vi "PipBoy_SearchLabVIEWs.vi"(8 "error in (no error)":errorcluster, 11 "PipBoyDataIn":T3) -> (0 "error out":errorcluster, 2 "LabVIEWEvents":T1[](array[typedef]), 3 "PipBoyDataOut":T3)   [LabVIEW 2014]
uses:
  ctls/PipBoy_PipBoyData.ctl
  ctls/PipBoy_ProcComm.ctl
  System.Windows.Forms
  ctls/PipBoy_PipBoyCommand.ctl
  ctls/PipBoy_Message.ctl
  modules/support/Message Queue/All Message Queues.ctl
  modules/support/Message Queue/Message Cluster.ctl
  ctls/PipBoy_FileConf.ctl
  ctls/PipBoy_PicComm.ctl
  ctls/PipBoy_GeneralParams.ctl
  ctls/PipBoy_Pages.ctl
  ctls/PipBoy_LabVIEWEvent.ctl
  ctls/PipBoy_DetectionType.ctl
  modules/support/Message Queue/Message Queue.lvlib
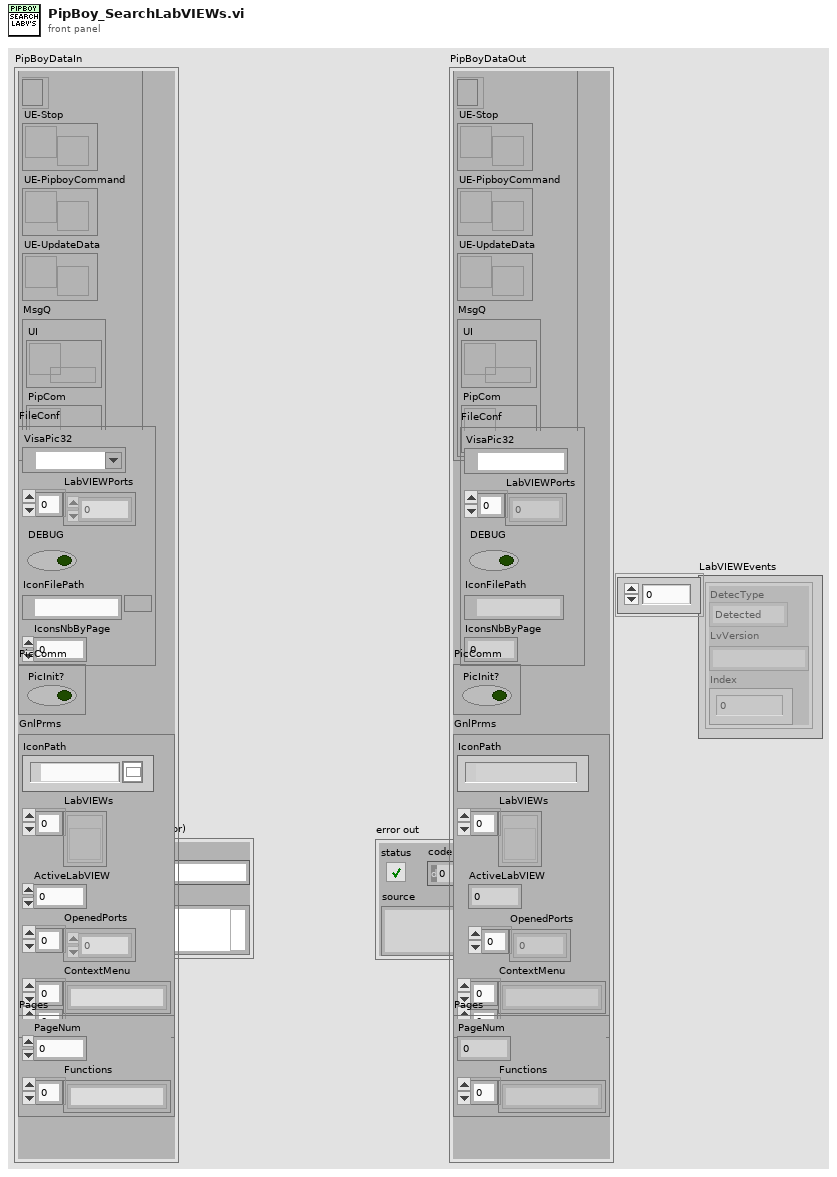
[diagram p1: front panel]
types:
  T1 = typedef "PipBoy_LabVIEWEvent.ctl" = cluster{"DetecType":T2, "LvVersion":string, "Index":i32}
  T2 = typedef "PipBoy_DetectionType.ctl" = enum16{"Detected", "Lost"}
  T3 = typedef "PipBoy_PipBoyData.ctl" = cluster{"ProcComm":T4, "FileConf":T6, "PicComm":T7, "GnlPrms":T8, "Pages":T9}
  T4 = typedef "PipBoy_ProcComm.ctl" = cluster{"NotifyIconRef":refnum<k24>, "UE-Stop":refnum<user-event>, "UE-PipboyCommand":refnum<user-event>, "UE-UpdateData":refnum<user-event>, "MsgQ":T5}
  T5 = typedef "Message Queue.lvlib/All Message Queues.ctl" = cluster{"UI":refnum<queue>, "PipCom":refnum<queue>}
  T6 = typedef "PipBoy_FileConf.ctl" = cluster{"VisaPic32":refnum<visa-resource-name>, "LabVIEWPorts":u16[], "DEBUG":bool, "IconFilePath":path, "IconsNbByPage":i32}
  T7 = typedef "PipBoy_PicComm.ctl" = cluster{"PicInit?":bool}
  T8 = typedef "PipBoy_GeneralParams.ctl" = cluster{"IconPath":path, "LabVIEWs":refnum<vi>[], "ActiveLabVIEW":i32, "OpenedPorts":u16[], "ContextMenu":string[][]}
  T9 = typedef "PipBoy_Pages.ctl" = cluster{"PageNum":i32, "Functions":string[]}
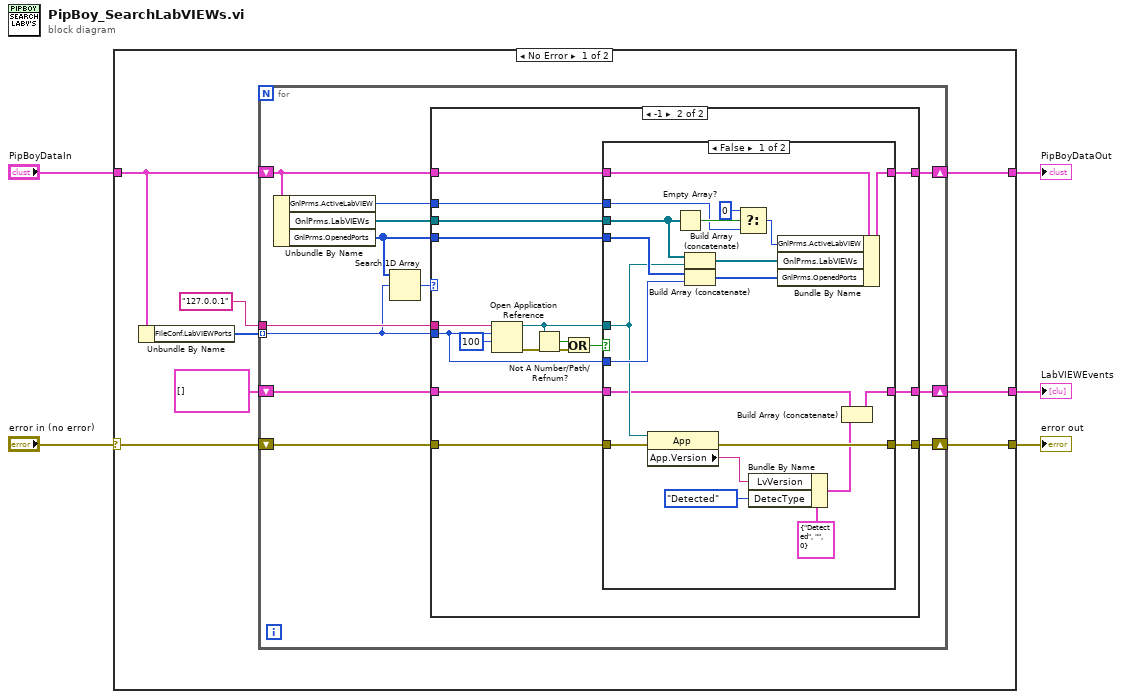
[diagram p0: block diagram]
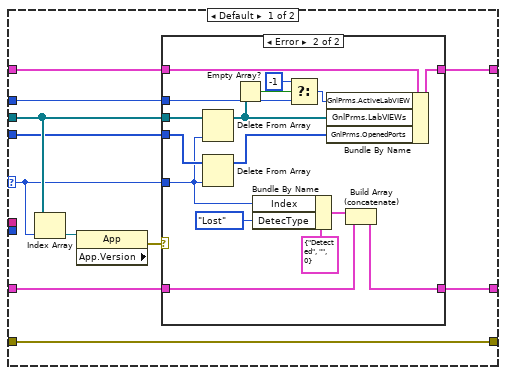
[diagram p2: hidden frame]
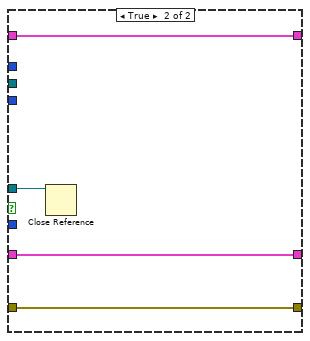
[diagram p4: hidden frame]
diagram:
  n1 = case shown="No Error" "error in (no error)" {
    selector: "error in (no error)" -> [w9 w96]
    tunnel: [w8 w96] -> w4
    tunnel: [w10 w95] -> w2
    tunnel: "PipBoyDataIn" -> [w11 w95]
    tunnel: [w6 _] -> w1
    frame No Error {
      n2 = Unbundle By Name(w11) -> ("FileConf.LabVIEWPorts"=w12:u16[])
      n3 = for {
        tunnel: "127.0.0.1" ("machine name (\"\":  open local reference)") -> [w25]
        tunnel: w12 -> [w22] mode=indexing
        shift-right: [w24] -> w10
        shift-left: w11 -> [w23]
        shift-right: [w16] -> w8
        shift-left: w9 -> [w17]
        shift-right: [w15] -> w6
        shift-left: T1[] [] -> [w14]
        n4 = Unbundle By Name(w23) -> ("GnlPrms.ActiveLabVIEW"=w18:i32, "GnlPrms.LabVIEWs"=w20:refnum<vi>[], "GnlPrms.OpenedPorts"=w19:u16[])
        n5 = Search 1D Array(1D array=w19, element=w22) -> (index of element=w21:i32)  [unwired: 1 in]
        n6 = case shown="-1" w21 {
          selector: w21 -> [w31 _]
          tunnel: w25 -> [_ w70]
          tunnel: [w34 w65] -> w24
          tunnel: w23 -> [w35 w64]
          tunnel: w22 -> [_ w63]
          tunnel: w20 -> [w32 w62]
          tunnel: w19 -> [w30 w61]
          tunnel: w18 -> [w29 w60]
          tunnel: w17 -> [w28 w59]
          tunnel: [w28 w58] -> w16
          tunnel: [w26 w57] -> w15
          tunnel: w14 -> [w27 w56]
          frame Default {
            n7 = Index Array(array=w32, index=w31) -> (element=w33:refnum<vi>)
            n8 = property class="App" props=["App.Version"](reference=w33) -> (error out=w36:errorcluster)  [unwired: 1 in, 2 out]
            n9 = case shown="Error" w36 {
              tunnel: w35 -> [w38 w54]
              tunnel: [w38 w53] -> w34
              tunnel: w32 -> [_ w52]
              tunnel: w31 -> [_ w39]
              tunnel: w30 -> [_ w51]
              tunnel: w29 -> [_ w47]
              tunnel: w27 -> [w37 w42]
              tunnel: [w37 w41] -> w26
              frame No Error {
              }
              frame Error {
                n10 = Delete From Array(array=w52, index=w39) -> (array with subset deleted=w49:refnum<vi>[])  [unwired: 1 in, 1 out]
                n11 = Delete From Array(array=w51, index=w39) -> (array with subset deleted=w50:u16[])  [unwired: 1 in, 1 out]
                n12 = Empty Array?(array=w49) -> (empty?=w48:bool)
                n13 = Bundle By Name(cluster=T1 {"DetecType"=enum."Detected", "LvVersion"="", "Index"=0} ("LabVIEWEvent"), "Index"=w39, "DetecType"=PipBoy_DetectionType."Lost") -> (w43:T1)
                n14 = Select(t=-1 ("GnlPrms.ActiveLabVIEW"), s=w48, f=w47) -> (s? t:f=w45:i32)
                n15 = Bundle By Name(cluster=w54, "GnlPrms.ActiveLabVIEW"=w45, "GnlPrms.LabVIEWs"=w49, "GnlPrms.OpenedPorts"=w50) -> (w53:T3)
                n16 = Build Array (concatenate)(w43, w42) -> (w41:T1[])
              }
            }
          }
          frame -1 {
            n17 = Open Application Reference(9:100 ("timeout ms (60000)"), 10:w63, 11:w70) -> (0:w68:errorcluster, 3:w66:refnum<vi>)  [unwired: 1 in]
            n18 = Not A Number/Path/Refnum?(number/path/refnum=w66) -> (NaN/Path/Refnum?=w69:bool)
            n19 = Or(x=w69, y=w68) -> (x .or. y?=w67:bool)
            n20 = case shown="False" w67 {
              tunnel: w66 -> [w79 w94]
              tunnel: w64 -> [w90 w93]
              tunnel: [w89 w93] -> w65
              tunnel: w63 -> [w88 _]
              tunnel: w62 -> [w83 _]
              tunnel: w61 -> [w86 _]
              tunnel: w60 -> [w81 _]
              tunnel: w59 -> [w78 w92]
              tunnel: [w77 w92] -> w58
              tunnel: [w71 w91] -> w57
              tunnel: w56 -> [w72 w91]
              frame False {
                n21 = property class="App"(reference=w79, error in=w78) -> (error out=w77:errorcluster, "App.Version"=w74:string)  [unwired: 1 out]
                n22 = Empty Array?(array=w83) -> (empty?=w82:bool)
                n23 = Build Array (concatenate)(w83, w79) -> (w85:refnum<vi>[])
                n24 = Build Array (concatenate)(w86, w88) -> (w87:u16[])
                n25 = Select(t=0 ("GnlPrms.ActiveLabVIEW"), s=w82, f=w81) -> (s? t:f=w80:i32)
                n26 = Bundle By Name(cluster=T1 {"DetecType"=enum."Detected", "LvVersion"="", "Index"=0} ("LabVIEWEvent"), "LvVersion"=w74, "DetecType"=PipBoy_DetectionType."Detected") -> (w73:T1)
                n27 = Bundle By Name(cluster=w90, "GnlPrms.ActiveLabVIEW"=w80, "GnlPrms.LabVIEWs"=w85, "GnlPrms.OpenedPorts"=w87) -> (w89:T3)
                n28 = Build Array (concatenate)(w72, w73) -> (w71:T1[])
              }
              frame True {
                n29 = Close Reference(reference=w94) -> ()  [unwired: 1 in, 1 out]
              }
            }
          }
        }
      }
    }
    frame Error {
    }
  }
  "error out" <- w4
  "PipBoyDataOut" <- w2
  "LabVIEWEvents" <- w1
